vi "Write Requirements Filepath.vi"(10 "File Path":path, 11 "Project in":refnum<class "RequirementsMap.lvclass">) -> (3 "Project out":refnum<class "RequirementsMap.lvclass">)   [LabVIEW 2021, in "Bananas.lvlib" / "RequirementsMap.lvclass"]
uses:
  RequirementsMap.lvclass
  RequirementsMap.lvclass/RequirementsMap.ctl
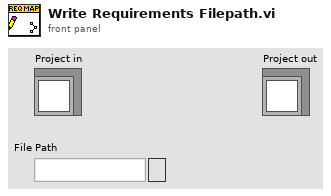
[diagram p1: front panel]
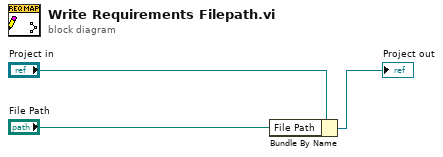
[diagram p0: block diagram]
diagram:
  n1 = Bundle By Name(cluster="Project in", "File Path"="File Path") -> (→"Project out":refnum<class "RequirementsMap.lvclass">)
